vi "SSFG_sharp.vi"() -> ()   [LabVIEW 2014]
uses:
  SSFG_States.ctl
  <vilib>/Utility/error.llb/DialogType.ctl
  <vilib>/DAQmx/write.llb/DAQmx Write (Analog Wfm 1Chan NSamp).vi
  <vilib>/DAQmx/read.llb/DAQmx Read (Analog Wfm 1Chan NSamp).vi
  <vilib>/DAQmx/create/channels.llb/DAQmx Create Channel (AO-Voltage-Basic).vi
  <vilib>/DAQmx/configure/timing.llb/DAQmx Timing (Sample Clock).vi
  <vilib>/DAQmx/create/channels.llb/DAQmx Create Channel (AI-Voltage-Basic).vi
  <vilib>/DAQmx/configure/trigger.llb/DAQmx Start Trigger (Digital Edge).vi
  <vilib>/DAQmx/miscellaneous.llb/DAQmx Fill In Error Info.vi
  <resource>/objmgr/daqmx.rc
  <vilib>/measure/NI_MABase.lvlib
panel:
  out "size(s)":i32
  in  "Physical Channel 2":tag="Dev1/ai0" caption="Physical Channel"
  in  "Sample Rate":dbl=10000.0 caption="Sample Rate (Hz)" format="%0.2f"
  out "Measurement":waveform(dbl)(graph)
  in  "stop 2":bool caption="stop"
  in  "Samples to Read":i32=1000
  out "cycle RMS":dbl format="%.2g"
  out "Numeric":i32
  out "Iterations":i32
  in  "Attenuation":dbl
  in  "Number of Samples/Cycle":dbl
  out "Generation":waveform(dbl)(graph)
  in  "stop":bool
  in  "Power Signal Parameters":T1={"Waveform Type"=0, "Amplitude"=1.0, "Frequency"=17.0} {"Frequency" format="%0.2p"; "Waveform Type" items=["Sine Wave", "Triangle Wave", "Square Wave", "Sawtooth Wave"]}
  out "Flicker":bool
  out "Swell":bool
  out "Sag":bool
  in  "Stop":bool
  in  "Update Rate":dbl=1000.0 format="%0.2f"
  in  "Generation":tag
  in  "Flicker":T2
  in  "Swell":cluster{"Swell_Time (sec)":dbl, "Swell":bool}
  in  "Sag":cluster{"Sag_Time (sec)":dbl, "Sag":bool}
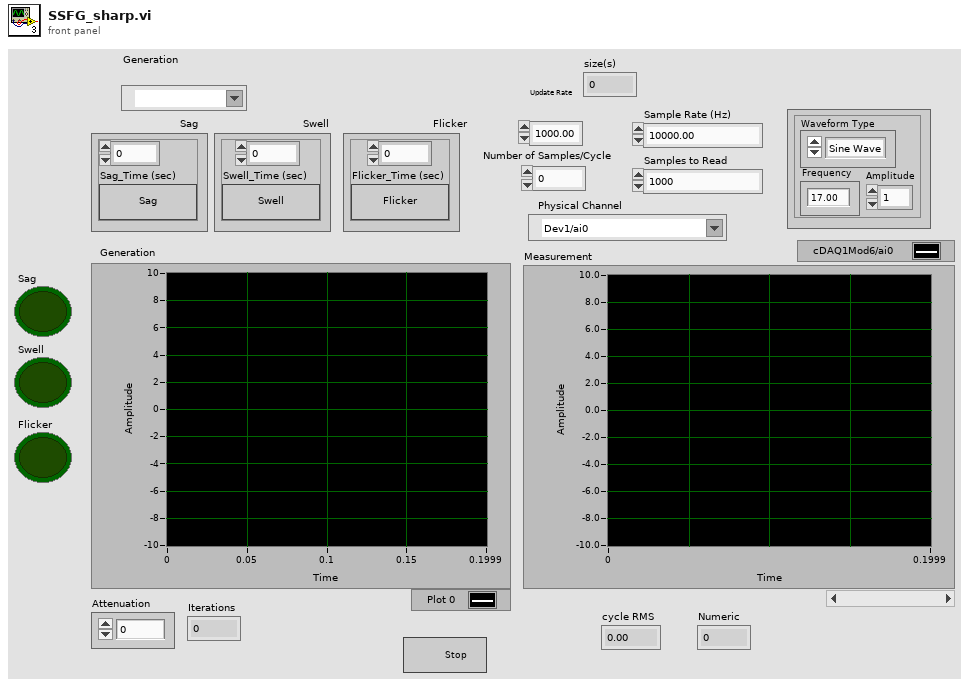
[diagram p1: front panel]
types:
  T1 = cluster{"Waveform Type":u16, "Amplitude":dbl, "Frequency":dbl}
  T2 = cluster{"Flicker_Time (sec)":dbl, "Flicker":bool}
  T3 = typedef "DialogType.ctl" = u16
  T4 = typedef "SSFG_States.ctl" = cluster{"State":string, "Disturbance_Time (sec)":dbl}
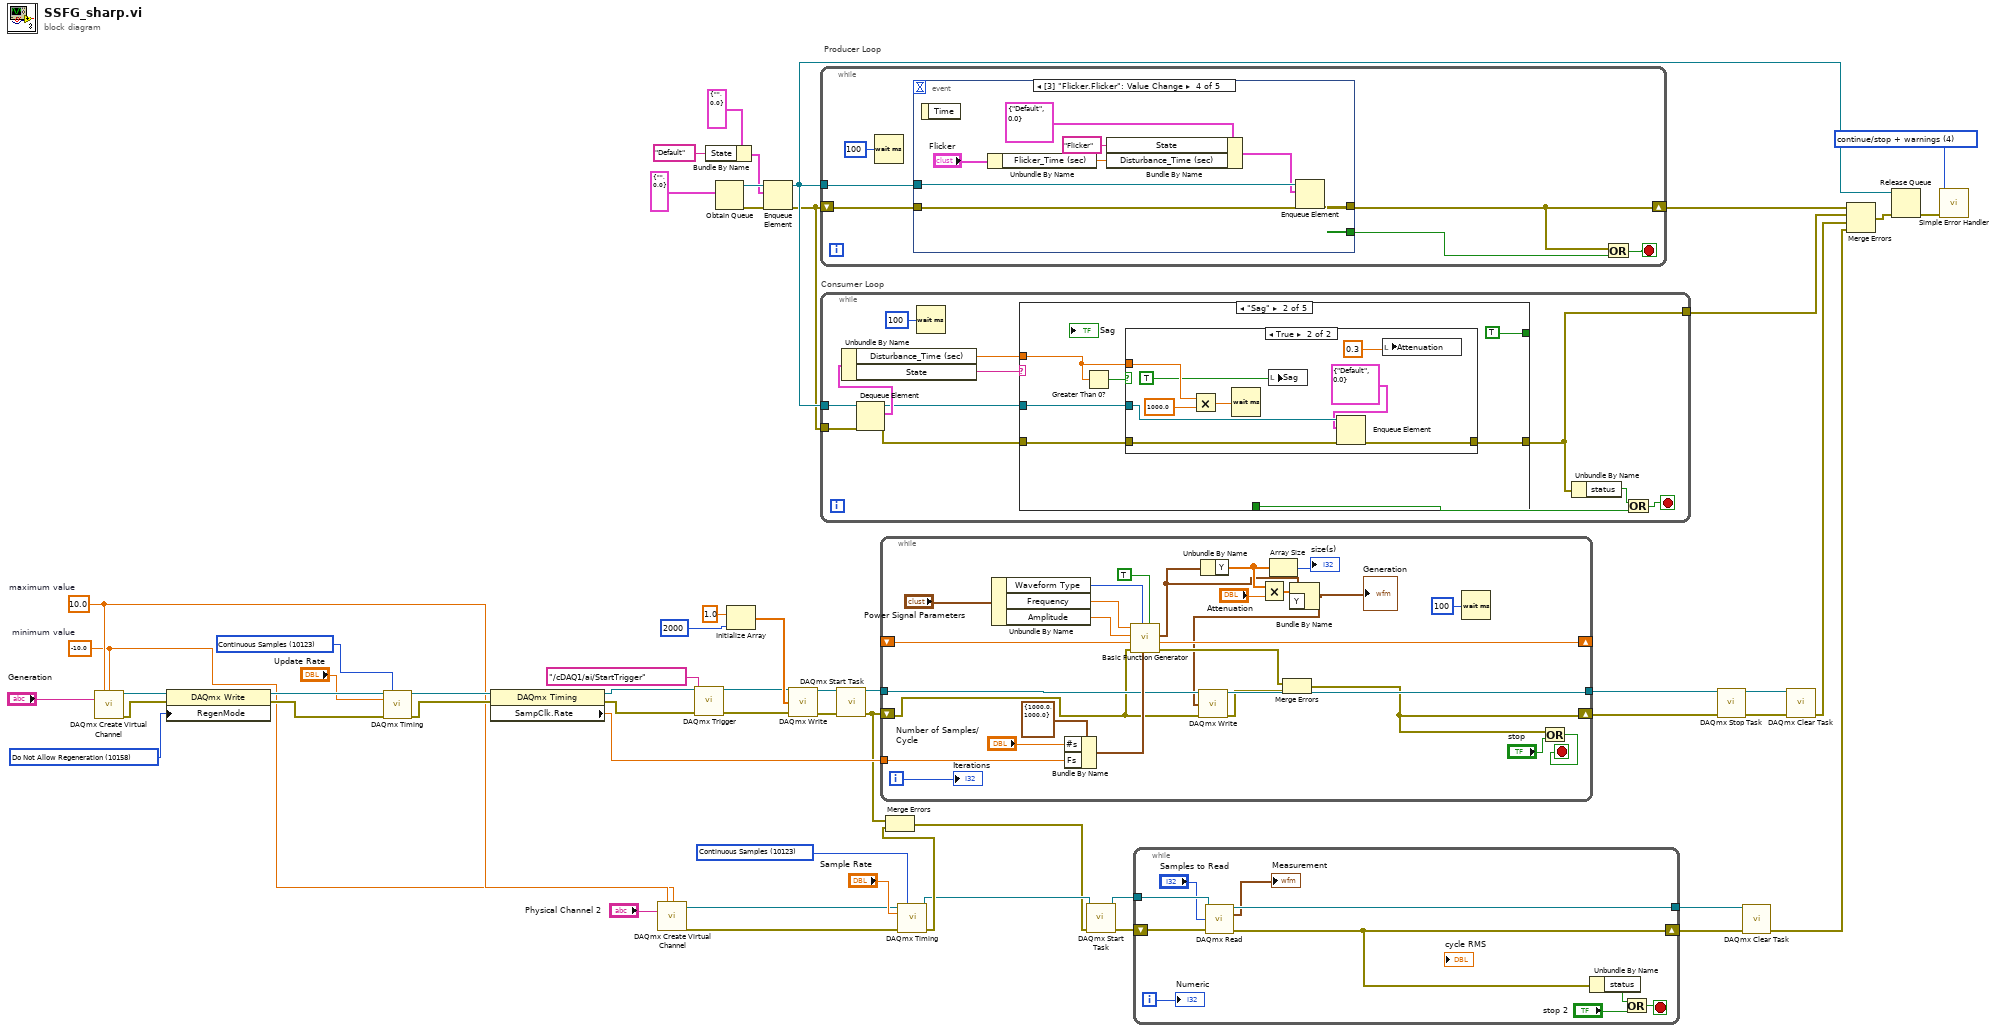
[diagram p0: block diagram]
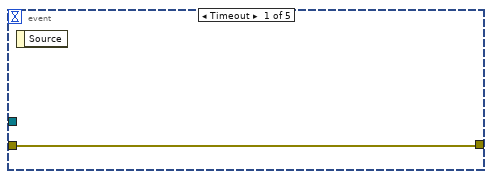
[diagram p2: hidden frame]
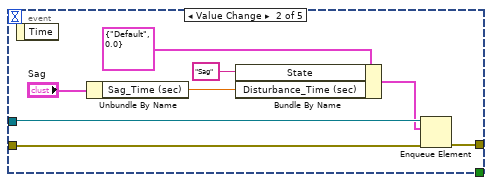
[diagram p3: hidden frame]
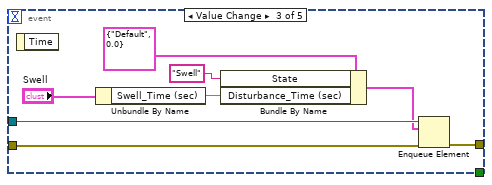
[diagram p4: hidden frame]
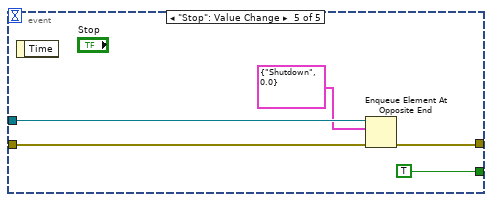
[diagram p5: hidden frame]
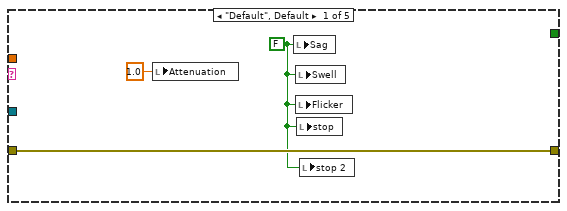
[diagram p6: hidden frame]
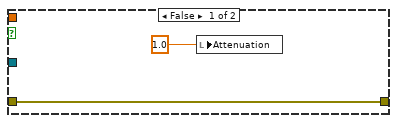
[diagram p7: hidden frame]
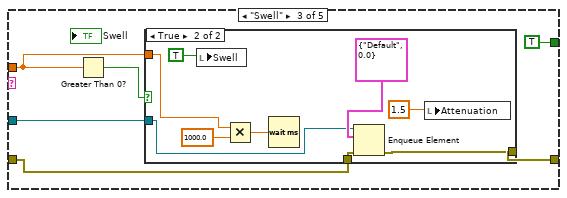
[diagram p8: hidden frame]
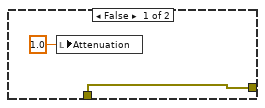
[diagram p9: hidden frame]
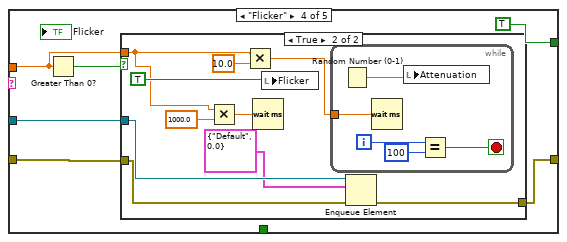
[diagram p10: hidden frame]
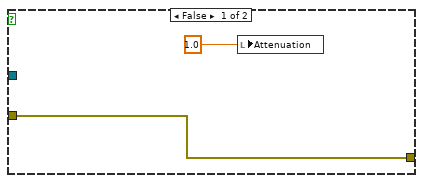
[diagram p11: hidden frame]
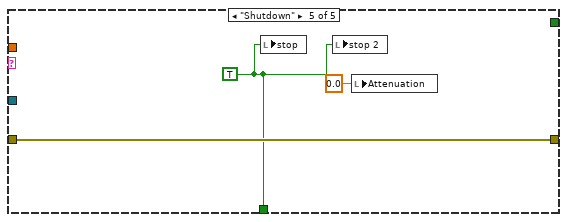
[diagram p12: hidden frame]
diagram:
  w1 = T3 4 items=["no dialog", "OK message", "continue or stop message", "OK message + warnings", "continue/stop + warnings"] ("type of dialog (OK msg:1)")
  w38 = 10123 items=["Finite Samples"=10178, "Continuous Samples"=10123] ("sample mode")
  w32 = 10.0  # maximum value
  w31 = -10.0  # minimum value
  w50 = 10123 items=["Finite Samples"=10178, "Continuous Samples"=10123, "Hardware Timed Single Point"=12522] ("sample mode")
  w51 = 10158 items=["Allow Regeneration"=10097, "Do Not Allow Regeneration"=10158] ("RegenMode")
  n1 = call-poly <vilib>:"DAQmx Create Virtual Channel.vi"("maximum value"=w32, "minimum value"=w31, "physical channels"="Generation") -> ("task out"=w55:refnum<k21>, "error out"=w53:errorcluster)  [unwired: 11 in]
  n2 = property class="DAQmx Write"(reference=w55, error in=w53, "RegenMode"=w51) -> (reference out=w54:refnum<k21>, error out=w52:errorcluster)
  n3 = call-poly <vilib>:"DAQmx Timing.vi"("task/channels in"=w54, "sample mode"=w50, "rate"="Update Rate", "error in"=w52) -> ("task out"=w44:refnum<k21>, "error out"=w43:errorcluster)  [unwired: 10 in]
  n4 = property class="DAQmx Timing"(reference=w44, error in=w43) -> (reference out=w27:refnum<k21>, error out=w25:errorcluster, "SampClk.Rate"=w47:dbl)
  n5 = call-poly <vilib>:"DAQmx Create Virtual Channel.vi"("maximum value"=w32, "minimum value"=w31, "physical channels"="Physical Channel 2") -> ("task out"=w34:refnum<k21>, "error out"=w33:errorcluster)  [unwired: 11 in]
  n6 = call-poly <vilib>:"DAQmx Trigger.vi"("task/channels in"=w27, "source"=tag "/cDAQ1/ai/StartTrigger", "error in"=w25) -> ("task out"=w26:refnum<k21>, "error out"=w24:errorcluster)  [unwired: 11 in]
  n7 = Bundle By Name(cluster=T4 {"State"="", "Disturbance_Time (sec)"=0.0}, "State"="Default") -> (w6:T4)
  n8 = Obtain Queue(element data type=T4 {"State"="", "Disturbance_Time (sec)"=0.0}) -> (queue out=w10:refnum<queue>, error out=w9:errorcluster)  [unwired: 4 in, 1 out]
  n9 = Initialize Array(1.0 ("element"), 2000 ("dimension size")) -> (w28:dbl[])
  n10 = Enqueue Element(queue=w10, element=w6, error in (no error)=w9) -> (queue out=w4:refnum<queue>, error out=w3:errorcluster)  [unwired: 1 in, 1 out]
  n11 = call-poly <vilib>:"DAQmx Write.vi"("task/channels in"=w26, "data"=w28, "error in"=w24) -> ("task out"=w22:refnum<k21>, "error out"=w19:errorcluster)  [unwired: 10 in, 1 out]
  n12 = while "Producer Loop" {
    tunnel: w4 -> [w61]
    shift-right: [w59] -> w12
    shift-left: w3 -> [w60]
    stop <- w62 stop-if-true
    n13 = Wait (ms)(milliseconds to wait=u32 100) -> ()  [unwired: 1 out]
    n14 = event shown="[3] \"Flicker.Flicker\": Value Change" {
      selector: _ -> [_ _ _ _ _]
      dyn-events: _ -> [_ _ _ _ _]
      timeout: _ -> [_ _ _ _ _]
      tunnel: w61 -> [_ w71 w79 w87 w92]
      tunnel: w60 -> [w63 w70 w78 w86 w91]
      tunnel: [w63 w69 w77 w85 w90] -> w59
      tunnel: [_ _ _ _ TRUE] -> w58
      event Timeout {
        n15 = event-data() -> ()  [unwired: 1 in, 1 out]
      }
      event "Sag.Sag": Value Change {
        n16 = event-data() -> ()  [unwired: 1 in, 1 out]
        n17 = Unbundle By Name("Sag") -> ("Sag_Time (sec)"=w66:dbl)
        n18 = Bundle By Name(cluster=T4 {"State"="Default", "Disturbance_Time (sec)"=0.0}, "State"="Sag", "Disturbance_Time (sec)"=w66) -> (w65:T4)
        n19 = Enqueue Element(queue=w71, element=w65, error in (no error)=w70) -> (error out=w69:errorcluster)  [unwired: 1 in, 2 out]
      }
      event "Swell.Swell": Value Change {
        n20 = event-data() -> ()  [unwired: 1 in, 1 out]
        n21 = Unbundle By Name("Swell") -> ("Swell_Time (sec)"=w75:dbl)
        n22 = Bundle By Name(cluster=T4 {"State"="Default", "Disturbance_Time (sec)"=0.0}, "State"="Swell", "Disturbance_Time (sec)"=w75) -> (w73:T4)
        n23 = Enqueue Element(queue=w79, element=w73, error in (no error)=w78) -> (error out=w77:errorcluster)  [unwired: 1 in, 2 out]
      }
      event "Flicker.Flicker": Value Change {
        n24 = event-data() -> ()  [unwired: 1 in, 1 out]
        n25 = Unbundle By Name("Flicker") -> ("Flicker_Time (sec)"=w82:dbl)
        n26 = Bundle By Name(cluster=T4 {"State"="Default", "Disturbance_Time (sec)"=0.0}, "State"="Flicker", "Disturbance_Time (sec)"=w82) -> (w81:T4)
        n27 = Enqueue Element(queue=w87, element=w81, error in (no error)=w86) -> (error out=w85:errorcluster)  [unwired: 1 in, 2 out]
      }
      event "Stop": Value Change {
        n28 = event-data() -> ()  [unwired: 1 in, 1 out]
        n29 = Enqueue Element At Opposite End(queue=w92, element=T4 {"State"="Shutdown", "Disturbance_Time (sec)"=0.0}, error in (no error)=w91) -> (error out=w90:errorcluster)  [unwired: 1 in, 2 out]
      }
    }
    n30 = Or(x=w59, y=w58) -> (x .or. y?=w62:bool)
  }
  n31 = while "Consumer Loop" {
    tunnel: [w97] -> w2
    tunnel: w4 -> [w102]
    tunnel: w3 -> [w101]
    stop <- w104 stop-if-true
    n32 = Dequeue Element(queue=w102, error in (no error)=w101) -> (queue out=w96:refnum<queue>, element=w100:T4, error out=w95:errorcluster)  [unwired: 1 in, 1 out]
    n33 = Unbundle By Name(w100) -> ("Disturbance_Time (sec)"=w94:dbl, "State"=w99:string)
    n34 = Wait (ms)(milliseconds to wait=u32 100) -> ()  [unwired: 1 out]
    n35 = case shown="\"Sag\"" w99 {
      tunnel: [_ _ _ _ w165] -> w98
      tunnel: w95 -> [w107 w110 w128 w145 w166]
      tunnel: [w107 w111 w127 w144 w166] -> w97
      tunnel: w96 -> [_ w109 w126 w143 _]
      tunnel: w94 -> [_ w112 w129 w146 _]
      tunnel: [_ TRUE TRUE TRUE _] -> _
      frame "Default", Default {
        w105 = FALSE ("Sag")
        n36 = local write "Attenuation"(1.0 ("Attenuation")) -> ()
        n37 = local write "Sag"(w105) -> ()
        n38 = local write "Swell"(w105) -> ()
        n39 = local write "Flicker"(w105) -> ()
        n40 = local write "stop"(w105) -> ()
        n41 = local write "stop 2"(w105) -> ()
      }
      frame "Sag" {
        n42 = Greater Than 0?(x=w112) -> (x > 0?=w113:bool)
        n43 = case shown="True" w113 {
          tunnel: w112 -> [_ w118]
          tunnel: [w114 w123] -> w111
          tunnel: w110 -> [w114 w122]
          tunnel: w109 -> [_ w121]
          frame False {
            n44 = local write "Attenuation"(1.0 ("y")) -> ()
          }
          frame True {
            n45 = Multiply(x=w118, y=1000.0) -> (x*y=w119:dbl)
            n46 = Wait (ms)(milliseconds to wait=w119) -> ()  [unwired: 1 out]
            n47 = local write "Sag"(TRUE ("Auto Reset")) -> ()
            n48 = Enqueue Element(queue=w121, element=T4 {"State"="Default", "Disturbance_Time (sec)"=0.0}, error in (no error)=w122) -> (error out=w123:errorcluster)  [unwired: 1 in, 2 out]
            n49 = local write "Attenuation"(0.3 ("y")) -> ()
          }
        }
      }
      frame "Swell" {
        n50 = Greater Than 0?(x=w129) -> (x > 0?=w130:bool)
        n51 = case shown="True" w130 {
          tunnel: w129 -> [_ w136]
          tunnel: w128 -> [w131 w140]
          tunnel: [w131 w139] -> w127
          tunnel: w126 -> [_ w134]
          frame False {
            n52 = local write "Attenuation"(1.0 ("y")) -> ()
          }
          frame True {
            n53 = local write "Swell"(TRUE ("Auto Reset")) -> ()
            n54 = Multiply(x=w136, y=1000.0) -> (x*y=w138:dbl)
            n55 = Wait (ms)(milliseconds to wait=w138) -> ()  [unwired: 1 out]
            n56 = Enqueue Element(queue=w134, element=T4 {"State"="Default", "Disturbance_Time (sec)"=0.0}, error in (no error)=w140) -> (error out=w139:errorcluster)  [unwired: 1 in, 2 out]
            n57 = local write "Attenuation"(1.5 ("y")) -> ()
          }
        }
      }
      frame "Flicker" {
        n58 = Greater Than 0?(x=w146) -> (x > 0?=w147:bool)
        n59 = case shown="True" w147 {
          tunnel: w146 -> [_ w151]
          tunnel: w145 -> [w148 w159]
          tunnel: [w148 w158] -> w144
          tunnel: w143 -> [_ w157]
          frame False {
            n60 = local write "Attenuation"(1.0 ("y")) -> ()
          }
          frame True {
            n61 = Multiply(x=w151, y=1000.0) -> (x*y=w155:dbl)
            n62 = Multiply(x=w151, y=10.0) -> (x*y=w150:dbl)
            n63 = Wait (ms)(milliseconds to wait=w155) -> ()  [unwired: 1 out]
            n64 = local write "Flicker"(TRUE ("Auto Reset")) -> ()
            n65 = while {
              tunnel: w150 -> [w164]
              i -> [w162]
              stop <- w161 stop-if-true
              n66 = Random Number (0-1)() -> (number: 0 to 1=w163:dbl)
              n67 = Wait (ms)(milliseconds to wait=w164) -> ()  [unwired: 1 out]
              n68 = local write "Attenuation"(w163) -> ()
              n69 = Equal?(x=w162, y=100) -> (x = y?=w161:bool)
            }
            n70 = Enqueue Element(queue=w157, element=T4 {"State"="Default", "Disturbance_Time (sec)"=0.0}, error in (no error)=w159) -> (error out=w158:errorcluster)  [unwired: 1 in, 2 out]
          }
        }
      }
      frame "Shutdown" {
        w165 = TRUE
        n71 = local write "stop"(w165) -> ()
        n72 = local write "stop 2"(w165) -> ()
        n73 = local write "Attenuation"(0.0 ("Attenuation")) -> ()
      }
    }
    n74 = Unbundle By Name(w97) -> ("status"=w103:bool)
    n75 = Or(x=w103, y=w98) -> (x .or. y?=w104:bool)
  }
  n76 = call <vilib>:"DAQmx Start Task.vi"("task/channels in"=w22, "error in"=w19) -> ("task out"=w21:refnum<k21>, "error out"=w18:errorcluster)  [unwired: 12 in]
  n77 = while {
    tunnel: [w193] -> w48
    tunnel: w21 -> [w180]
    tunnel: w47 -> [w186]
    shift-right: [w184] -> _
    shift-left: _ -> [w183]
    shift-right: [w173] -> w16
    shift-left: w18 -> [w179]
    i -> [w181]
    stop <- w177 stop-if-true
    n78 = Unbundle By Name("Power Signal Parameters") -> ("Waveform Type"=w192:u16, "Frequency"=w191:dbl, "Amplitude"=w190:dbl)
    n79 = Bundle By Name(cluster=cluster{"Fs":dbl, "#s":dbl} {"Fs"=1000.0, "#s"=1000.0} ("sampling info"), "#s"="Number of Samples/Cycle", "Fs"=w186) -> (w187:cluster{"Fs":dbl, "#s":dbl})
    n80 = call <vilib>:"Basic Function Generator.vi"("reset signal"=TRUE, "sampling info"=w187, "signal type"=w192, "error in (no error)"=w179, "phase"=w183, "amplitude"=w190, "frequency"=w191) -> ("error out"=w174:errorcluster, "phase out"=w184:dbl, "signal out"=w169:waveform(dbl))  [unwired: 2 in]
    n81 = Unbundle By Name(w169) -> ("Y"=w171:dbl[])
    n82 = Multiply(x=w171, y="Attenuation") -> (x*y=w170:dbl[])
    n83 = Array Size(array=w171) -> (size(s)=→"size(s)":i32)
    n84 = Bundle By Name(cluster=w169, "Y"=w170) -> (w168:waveform(dbl))
    "Generation" <- w168
    n85 = call-poly <vilib>:"DAQmx Write.vi"("task/channels in"=w180, "data"=w168, "error in"=w179) -> ("task out"=w193:refnum<k21>, "error out"=w175:errorcluster)  [unwired: 10 in, 1 out]
    n86 = Merge Errors(w174, w175) -> (w173:errorcluster)
    n87 = Wait (ms)(milliseconds to wait=u32 100) -> ()  [unwired: 1 out]
    n88 = Or(x=w173, y="stop") -> (x .or. y?=w177:bool)
    "Iterations" <- w181
  }
  n89 = call-poly <vilib>:"DAQmx Timing.vi"("task/channels in"=w34, "sample mode"=w38, "rate"="Sample Rate", "error in"=w33) -> ("task out"=w41:refnum<k21>, "error out"=w42:errorcluster)  [unwired: 10 in]
  n90 = Merge Errors(w18, w42) -> (w17:errorcluster)
  n91 = call <vilib>:"DAQmx Start Task.vi"("task/channels in"=w41, "error in"=w17) -> ("task out"=w35:refnum<k21>, "error out"=w20:errorcluster)  [unwired: 12 in]
  n92 = while {
    tunnel: w35 -> [w203]
    tunnel: [w202] -> w36
    shift-right: [w199] -> w39
    shift-left: w20 -> [w204]
    i -> [w200]
    stop <- w196 stop-if-true
    n93 = call-poly <vilib>:"DAQmx Read.vi"("task/channels in"=w203, "number of samples per channel"="Samples to Read", "error in"=w204) -> ("task out"=w202:refnum<k21>, "data"=→"Measurement":waveform(dbl), "error out"=w199:errorcluster)  [unwired: 10 in]
    n94 = Unbundle By Name(w199) -> ("status"=w197:bool)
    n95 = Or(x=w197, y="stop 2") -> (x .or. y?=w196:bool)
    "Numeric" <- w200
  }
  n96 = call <vilib>:"DAQmx Stop Task.vi"("task/channels in"=w48, "error in"=w16) -> ("task out"=w46:refnum<k21>, "error out"=w45:errorcluster)  [unwired: 12 in]
  n97 = call <vilib>:"DAQmx Clear Task.vi"("task in"=w36, "error in"=w39) -> ("error out"=w15:errorcluster)  [unwired: 13 in]
  n98 = call <vilib>:"DAQmx Clear Task.vi"("task in"=w46, "error in"=w45) -> ("error out"=w14:errorcluster)  [unwired: 13 in]
  n99 = Merge Errors(w12, w2, w14, w15) -> (w11:errorcluster)
  n100 = Release Queue(queue=w4, error in (no error)=w11) -> (error out=w13:errorcluster)  [unwired: 1 in, 2 out]
  n101 = call <vilib>:"Simple Error Handler.vi"("type of dialog (OK msg:1)"=w1, "error in (no error)"=w13) -> ()  [unwired: 3 in, 5 out]
